vi "Write AO_index.vi"(9 "Reg":string, 10 "EnumsAO":string[](array[string]), 11 "bronkhorst_reg in":refnum<class "bronkhorst_reg_2.lvclass">) -> (2 "Find":bool, 3 "bronkhorst_reg out":refnum<class "bronkhorst_reg_2.lvclass">)   [LabVIEW 2019, in "control.lvlib" / "bronkhorst_reg_2.lvclass"]
uses:
  bronkhorst_reg_2.lvclass
  bronkhorst_reg_2.lvclass/bronkhorst_reg_2.ctl
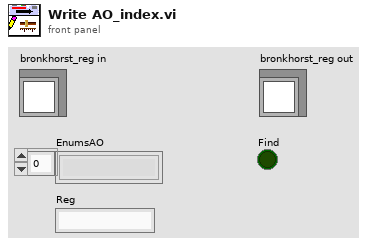
[diagram p1: front panel]
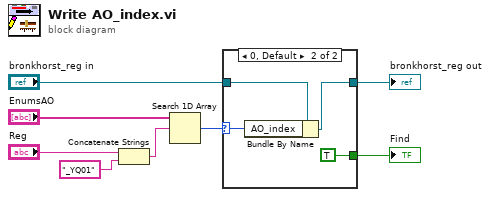
[diagram p0: block diagram]
diagram:
  n1 = Concatenate Strings("Reg", "_YQ01" ("string")) -> (w7:string)
  n2 = Search 1D Array(1D array="EnumsAO", element=w7) -> (index of element=w4:i32)  [unwired: 1 in]
  n3 = case shown="0, Default" w4 {
    selector: w4 -> [_ w11]
    tunnel: "bronkhorst_reg in" -> [w9 w13]
    tunnel: [w9 w12] -> w1
    tunnel: [_ TRUE] -> w3
    frame -1 {
    }
    frame 0, Default {
      n4 = Bundle By Name(cluster=w13, "AO_index"=w11) -> (w12:refnum<class "bronkhorst_reg_2.lvclass">)
    }
  }
  "bronkhorst_reg out" <- w1
  "Find" <- w3
